vi "dsbsc.vi"() -> ()   [LabVIEW 2016]
uses:
  <vilib>/measure/maspectr.llb/FFT Spectrum (Mag-Phase) for N Chan.vi
  <vilib>/measure/NI_MAPro.lvlib
panel:
  out "Output\n Graph 4":cluster{"f0":dbl, "df":dbl, "magnitude":dbl[]}[](graph)
  out "msg\n Graph 3":dynamicdata(graph)
  out "carrier\n Graph 2":dynamicdata(graph)
  out "Output\n Graph":dynamicdata(graph)
  in  "Carrier Frequency 2":dbl(knob)=10.1 caption="Frequency" scale=0.0..10000.0
  in  "MessageFrequency":dbl(knob)=10.1 caption="Frequency" scale=0.0..10.0
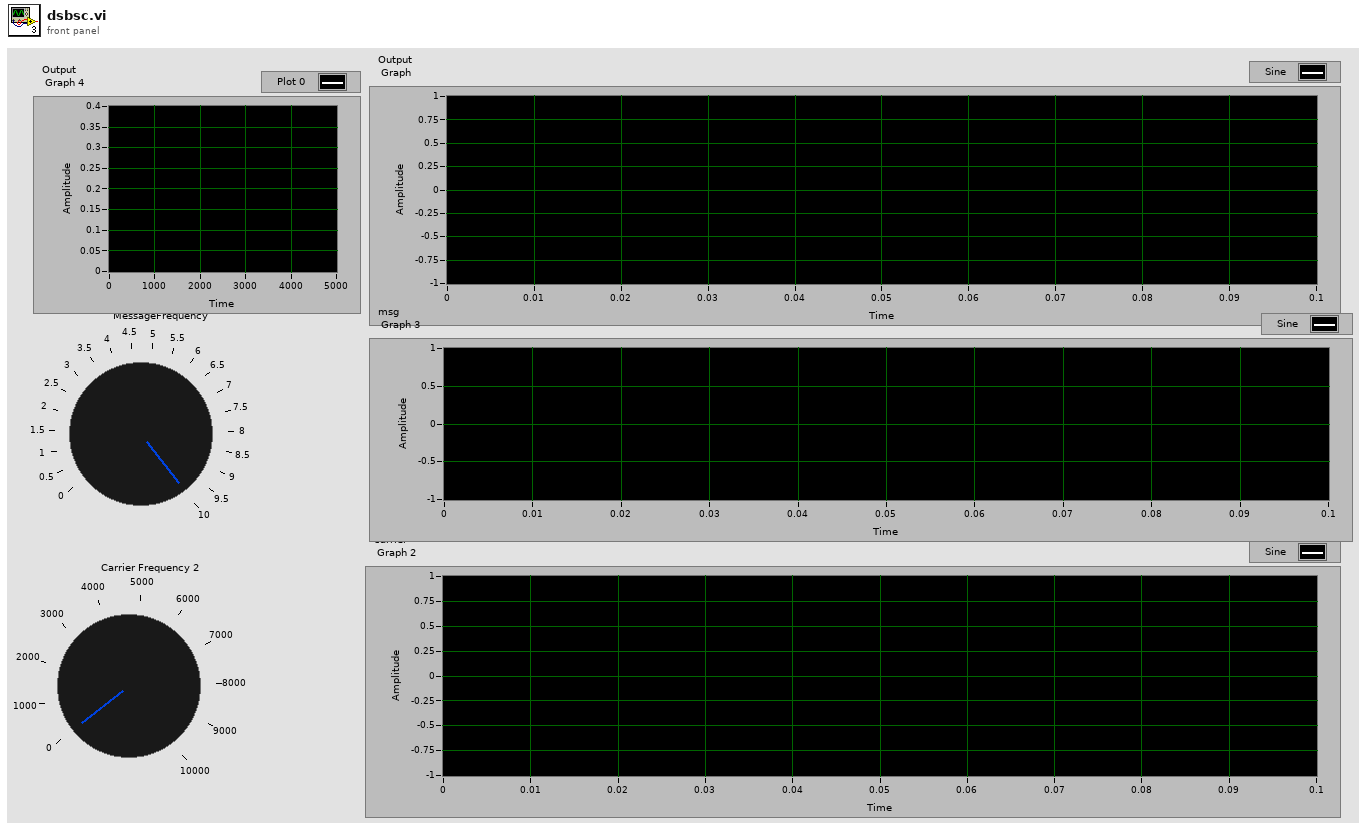
[diagram p1: front panel]
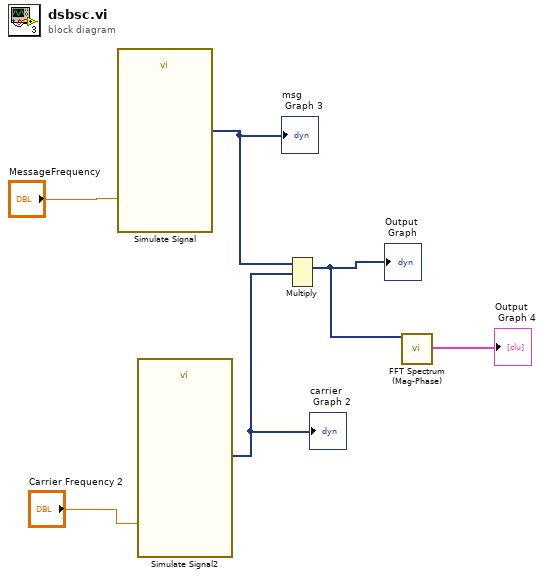
[diagram p0: block diagram]
diagram:
  n1 = call "Simulate Signal"("Frequency"="MessageFrequency") -> ("Sine"=w3:dynamicdata)  [unwired: 13 in, 1 out]
  "msg\n Graph 3" <- w3
  n2 = call "Simulate Signal2"("Frequency"="Carrier Frequency 2") -> ("Sine"=w4:dynamicdata)  [unwired: 13 in, 1 out]
  "carrier\n Graph 2" <- w4
  n3 = Multiply(1:w4, 2:w3) -> (0:w2:dynamicdata)  [unwired: 1 in, 1 out]
  "Output\n Graph" <- w2
  n4 = call-poly <vilib>:"FFT Spectrum (Mag-Phase).vi"("time signals"=w2) -> ("magnitudes"=→"Output\n Graph 4":cluster{"f0":dbl, "df":dbl, "magnitude":dbl[]}[])  [unwired: 6 in, 4 out]
